vi "Stop Core.vi"(10 "final error code":i32, 11 "Keypad in":refnum<class "Keypad.lvclass">) -> (3 "Keypad out":refnum<class "Keypad.lvclass">)   [LabVIEW 2020, in "Keypad.lvlib" / "Keypad.lvclass"]
doc: "(<B>Filename</B>: Actor Framework.lvlib:Actor.lvclass:Stop Core.vi)\n\nDefines what the actor does before it stops. Use the <B>final error code</B> input to determine whether the actor shut down in response to an error.\n\nBy default, this method does nothing. A descendant class may override it to define behavior, such as shutting down any processes the actor initiated in its override of the Actor Core method."
uses:
  Keypad.lvclass
  <vilib>/ni/Actors/State Actor/State Actor/State Actor.lvclass
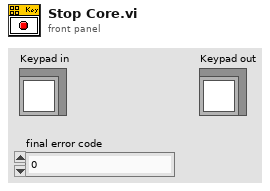
[diagram p1: front panel]
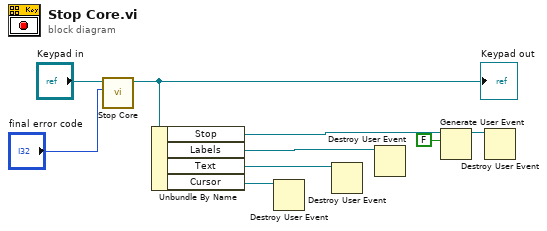
[diagram p0: block diagram]
diagram:
  n1 = call-parent "Stop Core.vi"("final error code"="final error code", "Actor in"="Keypad in") -> ("Actor out"=w7:refnum<class "Keypad.lvclass">)  [unwired: 9 in]
  "Keypad out" <- w7
  n2 = Unbundle By Name(w7) -> ("Stop"=w6:refnum<user-event>, "Labels"=w4:refnum<user-event>, "Text"=w3:refnum<user-event>, "Cursor"=w2:refnum<user-event>)
  n3 = Destroy User Event(user event=w2) -> ()  [unwired: 1 in, 1 out]
  n4 = Destroy User Event(user event=w3) -> ()  [unwired: 1 in, 1 out]
  n5 = Destroy User Event(user event=w4) -> ()  [unwired: 1 in, 1 out]
  n6 = Generate User Event(user event=w6, event data cluster=FALSE ("event data")) -> (user event out=w1:refnum<user-event>)  [unwired: 2 in, 1 out]
  n7 = Destroy User Event(user event=w1) -> ()  [unwired: 1 in, 1 out]
